vi "gating.vi"(10 "Cluster":T1, 11 "Array in":dbl[][](array[numeric])) -> (2 "Array":bool[](array[boolean]), 3 "Array out":dbl[][](array[numeric]))   [LabVIEW 2018]
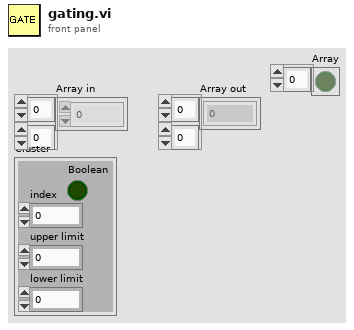
[diagram p1: front panel]
types:
  T1 = cluster{"index":i32, "upper limit":dbl, "lower limit":dbl, "Boolean":bool}
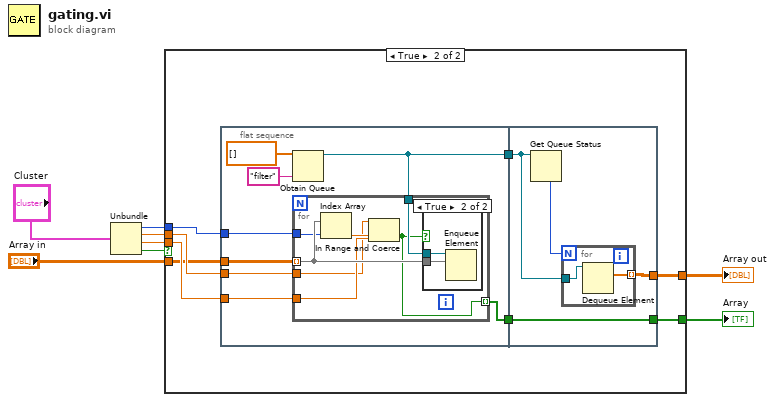
[diagram p0: block diagram]
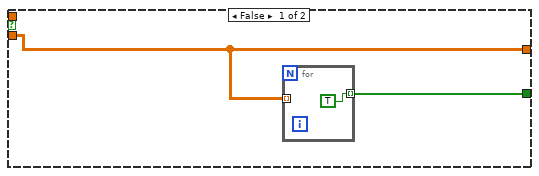
[diagram p2: hidden frame]
diagram:
  n1 = Unbundle("Cluster") -> ("index"=w8:i32, "upper limit"=w6:dbl, "lower limit"=w7:dbl, "Boolean"=w1:bool)
  n2 = case shown="True" w1 {
    tunnel: w8 -> [_ w17]
    tunnel: w7 -> [_ w16]
    tunnel: w6 -> [_ w15]
    tunnel: [w10 w14] -> w4
    tunnel: "Array in" -> [w10 w13]
    tunnel: [w9 w12] -> w2
    frame False {
      n3 = for {
        tunnel: w10 -> [_] mode=indexing
        tunnel: [TRUE] -> w9 mode=indexing
      }
    }
    frame True {
      n4 = flat-sequence {
        tunnel: w13 -> [w27]
        tunnel: [w24] -> w19
        tunnel: w17 -> [w23]
        tunnel: w16 -> [w22]
        tunnel: w15 -> [w21]
        tunnel: [w20] -> w18
        tunnel: w19 -> [w39]
        tunnel: [w38] -> w14
        tunnel: [w37] -> w12
        tunnel: w18 -> [w37]
        frame #0 {
          n5 = Obtain Queue(name (unnamed)="filter", element data type=dbl[] []) -> (queue out=w24:refnum<queue>)  [unwired: 3 in, 2 out]
          n6 = for {
            tunnel: w27 -> [w33] mode=indexing
            tunnel: w24 -> [w34]
            tunnel: w23 -> [w31]
            tunnel: w22 -> [w30]
            tunnel: w21 -> [w29]
            tunnel: [w28] -> w20 mode=indexing
            n7 = Index Array(array=w33, index=w31) -> (element=w32:dbl)
            n8 = In Range and Coerce(upper limit=w29, x=w32, lower limit=w30) -> (In Range?=w28:bool)  [unwired: 1 out]
            n9 = case shown="True" w28 {
              tunnel: w34 -> [_ w36]
              tunnel: w33 -> [_ w35]
              frame False {
              }
              frame True {
                n10 = Enqueue Element(queue=w36, element=w35) -> ()  [unwired: 2 in, 3 out]
              }
            }
          }
        }
        frame #1 {
          n11 = Get Queue Status(queue=w39) -> (# elements in queue=w40:i32)  [unwired: 2 in, 7 out]
          n12 = for {
            N: w40 -> [_]
            tunnel: w39 -> [w42]
            tunnel: [w41] -> w38 mode=indexing
            n13 = Dequeue Element(queue=w42) -> (element=w41:dbl[])  [unwired: 2 in, 3 out]
          }
        }
      }
    }
  }
  "Array out" <- w4
  "Array" <- w2
